vi "Add Rows (String).vi"(7 "image path":path, 8 "error in (no error)":errorcluster, 9 "String Data":string[][](array[string]), 11 "DataTable in":refnum<class "DataTable.lvclass">) -> (0 "error out":errorcluster, 3 "DataTable out":refnum<class "DataTable.lvclass">)   [LabVIEW 2020, in "DataGrid.lvlib" / "DataTable.lvclass"]
doc: "This allows any number of rows to be added to the datatable. The data must match the columns defined for the grid."
uses:
  DataTable.lvclass
  DataTable.lvclass/DataTable.ctl
  System.Data
  GridColumn/GridColumn.lvclass/GridColumn.ctl
  GridColumn/Read datatype.vi
  GridColumn/Read Params.vi
  GridColumn/Read Name.vi
  GridColumn/GridColumn.lvclass
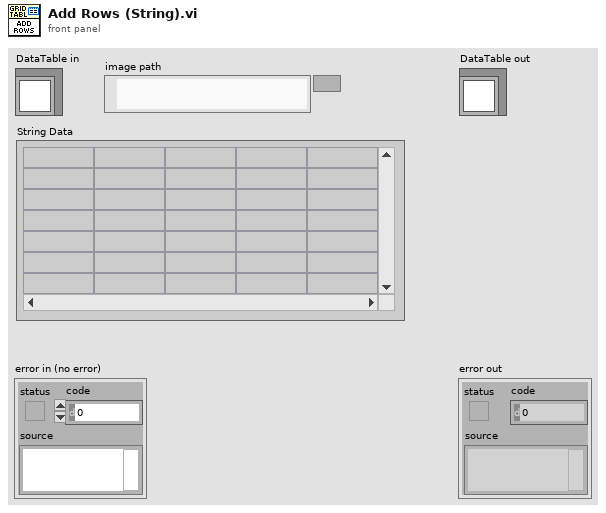
[diagram p1: front panel]
types:
  T1 = typedef "DataGrid.lvlib/GridColumn.lvclass/ColumnType.ctl" = enum16{"string", "image", "check", "numeric", "timestamp", "button", "combo", "link"}
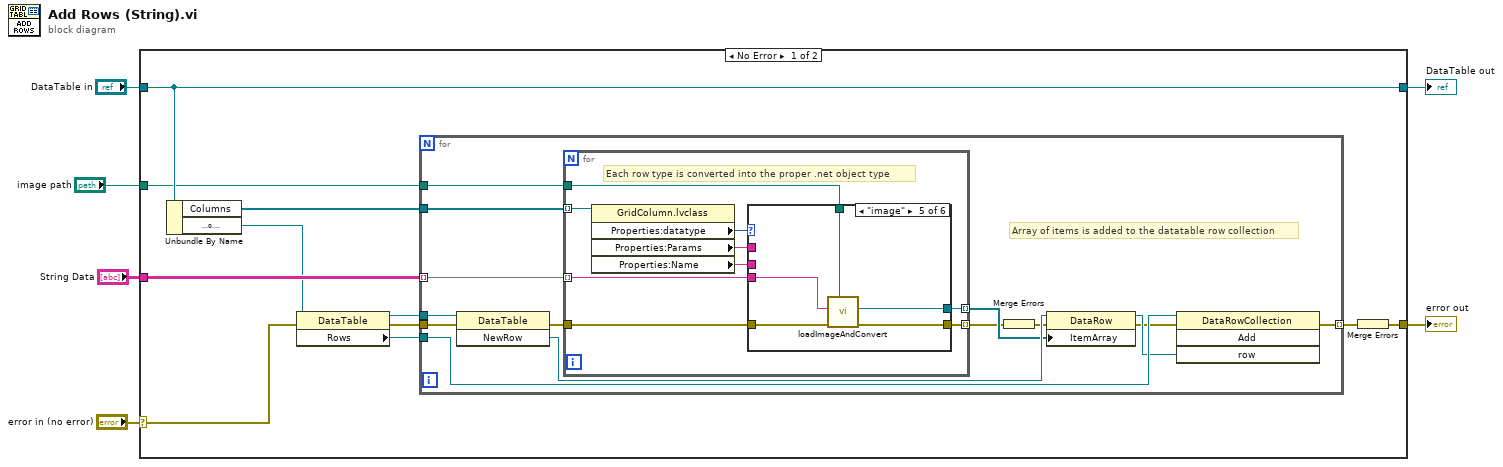
[diagram p0: block diagram]
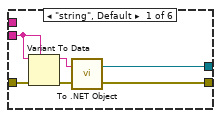
[diagram p2: hidden frame]
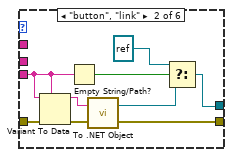
[diagram p3: hidden frame]
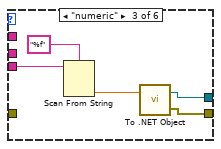
[diagram p4: hidden frame]
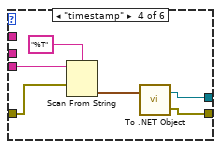
[diagram p5: hidden frame]
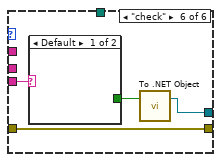
[diagram p6: hidden frame]
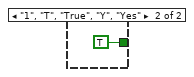
[diagram p7: hidden frame]
diagram:
  n1 = case shown="No Error" "error in (no error)" {
    selector: "error in (no error)" -> [w13 w77]
    tunnel: [w14 w78] -> w4
    tunnel: "DataTable in" -> [w14 w78]
    tunnel: "String Data" -> [w12 _]
    tunnel: [w9 w77] -> w2
    tunnel: "image path" -> [w7 _]
    frame No Error {
      n2 = Unbundle By Name(w14) -> ("Columns"=w8:refnum<class "GridColumn.lvclass">[], "DataTable"=w11:refnum<k24>)
      n3 = property class="DataTable"(reference=w11, error in=w13) -> (reference out=w10:refnum<k24>, error out=w17:errorcluster, "Rows"=w16:refnum<k24>)
      n4 = for {
        tunnel: w16 -> [w30]
        tunnel: w10 -> [w31]
        tunnel: [w29] -> w15 mode=indexing
        tunnel: w12 -> [w28] mode=indexing
        tunnel: w17 -> [w20]
        tunnel: w8 -> [w19]
        tunnel: w7 -> [w18]
        # "Array of items is added to the datatable row collection"
        n5 = invoke class="DataTable" method="NewRow"(reference=w31, error in=w20) -> (error out=w27:errorcluster, "NewRow"=w26:refnum<k24>)  [unwired: 1 in, 1 out]
        n6 = for {
          tunnel: w28 -> [w40] mode=indexing
          tunnel: [w39] -> w24 mode=indexing
          tunnel: w27 -> [w38]
          tunnel: [w37] -> w23 mode=indexing
          tunnel: w19 -> [w36] mode=indexing
          tunnel: w18 -> [w32]
          # "Each row type is converted into the proper .net object type"
          n7 = property class="GridColumn.lvclass"(reference=w36) -> ("Properties:datatype"=w35:T1, "Properties:Params"=w34:string, "Properties:Name"=w33:string)  [unwired: 1 in, 2 out]
          n8 = case shown="\"image\"" w35 {
            tunnel: w40 -> [w42 w51 w58 w64 w71 w73]
            tunnel: [w41 w48 w59 w65 w70 w74] -> w39
            tunnel: w38 -> [w45 w54 _ w62 w69 w75]
            tunnel: [w43 w52 w60 w66 w68 w75] -> w37
            tunnel: w34 -> [_ _ _ _ _ _]
            tunnel: w33 -> [_ _ _ _ _ _]
            tunnel: w32 -> [_ _ _ _ w67 _]
            frame "string", Default {
              n9 = Variant To Data(error in=w45, type=w42, Variant=w42) -> (data=w46:string, error out=w44:errorcluster)
              n10 = call <vilib>:"To .NET Object.vi"("error in (no error)"=w44, "anything"=w46) -> ("error out"=w43:errorcluster, ".NET object"=w41:refnum<k24>)
            }
            frame "button", "link" {
              n11 = Variant To Data(error in=w54, type=w51, Variant=w51) -> (data=w55:string, error out=w53:errorcluster)
              n12 = Empty String/Path?(string/path=w51) -> (empty?=w50:bool)
              n13 = call <vilib>:"To .NET Object.vi"("error in (no error)"=w53, "anything"=w55) -> ("error out"=w52:errorcluster, ".NET object"=w49:refnum<k24>)
              n14 = Select(t=refnum<k24> refnum, s=w50, f=w49) -> (s? t:f=w48:refnum<k24>)
            }
            frame "numeric" {
              n15 = Scan From String(format string="%f", input string=w58) -> (output 1=w56:dbl)  [unwired: 3 in, 3 out]
              n16 = call <vilib>:"To .NET Object.vi"("anything"=w56) -> ("error out"=w60:errorcluster, ".NET object"=w59:refnum<k24>)  [unwired: 1 in]
            }
            frame "timestamp" {
              n17 = Scan From String(format string="%T", input string=w64, error in=w62) -> (output 1=w61:timestamp)  [unwired: 2 in, 3 out]
              n18 = call <vilib>:"To .NET Object.vi"("anything"=w61) -> ("error out"=w66:errorcluster, ".NET object"=w65:refnum<k24>)  [unwired: 1 in]
            }
            frame "image" {
              n19 = call "loadImageAndConvert.vi"("image path"=w67, "error in (no error)"=w69, "name or relative path"=w71) -> ("error out"=w68:errorcluster, ".NET object"=w70:refnum<k24>)  [unwired: 7 in]
            }
            frame "check" {
              n20 = case shown="Default" w73 {
                tunnel: [_ TRUE] -> w72
                frame Default {
                }
                frame "1", "T", "True", "Y", "Yes" {
                }
              }
              n21 = call <vilib>:"To .NET Object.vi"("anything"=w72) -> (".NET object"=w74:refnum<k24>)  [unwired: 1 in, 1 out]
            }
          }
        }
        n22 = Merge Errors(w23) -> (w22:errorcluster)
        n23 = property class="DataRow"(reference=w26, error in=w22, "ItemArray"=w24) -> (reference out=w25:refnum<k24>, error out=w21:errorcluster)
        n24 = invoke class="DataRowCollection" method="Add"(reference=w30, error in=w21, "row"=w25) -> (error out=w29:errorcluster)  [unwired: 1 in, 3 out]
      }
      n25 = Merge Errors(w15) -> (w9:errorcluster)
    }
    frame Error {
    }
  }
  "error out" <- w2
  "DataTable out" <- w4
